vi "NI-XNET Monitor Init.vi"(8 "Error In":errorcluster, 10 "Parameters":variant, 11 "Data Access Engine in":refnum<class "Data Access Engine.lvclass">) -> (0 "Error Out":errorcluster, 3 "Process  Data Out":T1, 4 "Async Loop Rate (s)":dbl)   [LabVIEW 2018, in "NI-XNET Monitor Engine.lvlib"]
uses:
  NI-XNET Monitor Engine.lvlib
  <vilib>/NI/NIVS Inline Async API/_Data Access Engine/Data Access Engine/Data Access Engine.lvclass
  typedefs/RTMonitorRefnums.ctl
  typedefs/CANBus.Settings.ctl
  Bus Load/CANBus/CANBus_Load_Calculator.lvclass
  <vilib>/NI/NIVS Inline Async API/_Data Access Engine/Data Access Engine/Types/Write.DVR.ctl
  <vilib>/NI/NIVS Inline Async API/_Data Access Engine/Access Type Classes/Write/Write.lvclass
  Shared/Compiled.Data.ctl
  Shared/BusLoad.Settings.ctl
  <vilib>/NI/NIVS Inline Async API/_Data Access Engine/Data Access Engine/Methods/Write.Lookup.vi
  Shared/NI-XNET Monitor Shared.lvlib
  <vilib>/NI Veristand/Custom Device Tools/Custom Device Utility Library/Custom Device Utility Library.lvlib
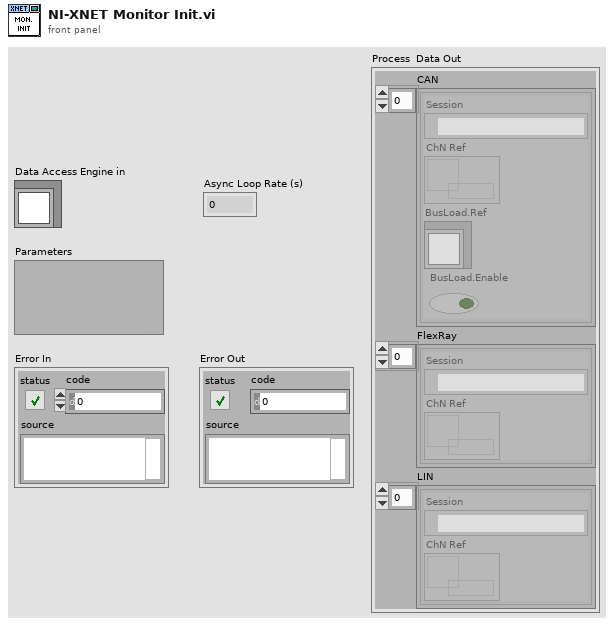
[diagram p1: front panel]
types:
  T1 = typedef "NI-XNET Monitor Engine.lvlib/RTMonitorRefnums.ctl" = cluster{"CAN":T2[], "FlexRay":cluster{"Session":refnum<k21>, "ChN Ref":T3}[], "LIN":cluster{"Session":refnum<k21>, "ChN Ref":T3}[]}
  T2 = typedef "NI-XNET Monitor Engine.lvlib/CANBus.Settings.ctl" = cluster{"Session":refnum<k21>, "ChN Ref":T3, "BusLoad.Ref":refnum<class "CANBus_Load_Calculator.lvclass">, "BusLoad.Enable":bool}
  T3 = typedef "Data Access Engine.lvlib/Data Access Engine.lvclass/Write.DVR.ctl" = refnum<data-value>
  T4 = typedef "NI-XNET Monitor Shared.lvlib/Compiled.Data.ctl" = cluster{"CAN":string[], "FlexRay":string[], "LIN":string[], "Async Loop Rate (s)":dbl, "CAN.BusLoad.Settings":T5[]}
  T5 = typedef "NI-XNET Monitor Shared.lvlib/BusLoad.Settings.ctl" = cluster{"BusLoad.Disable":bool, "BusLoad.Periodms":u32}
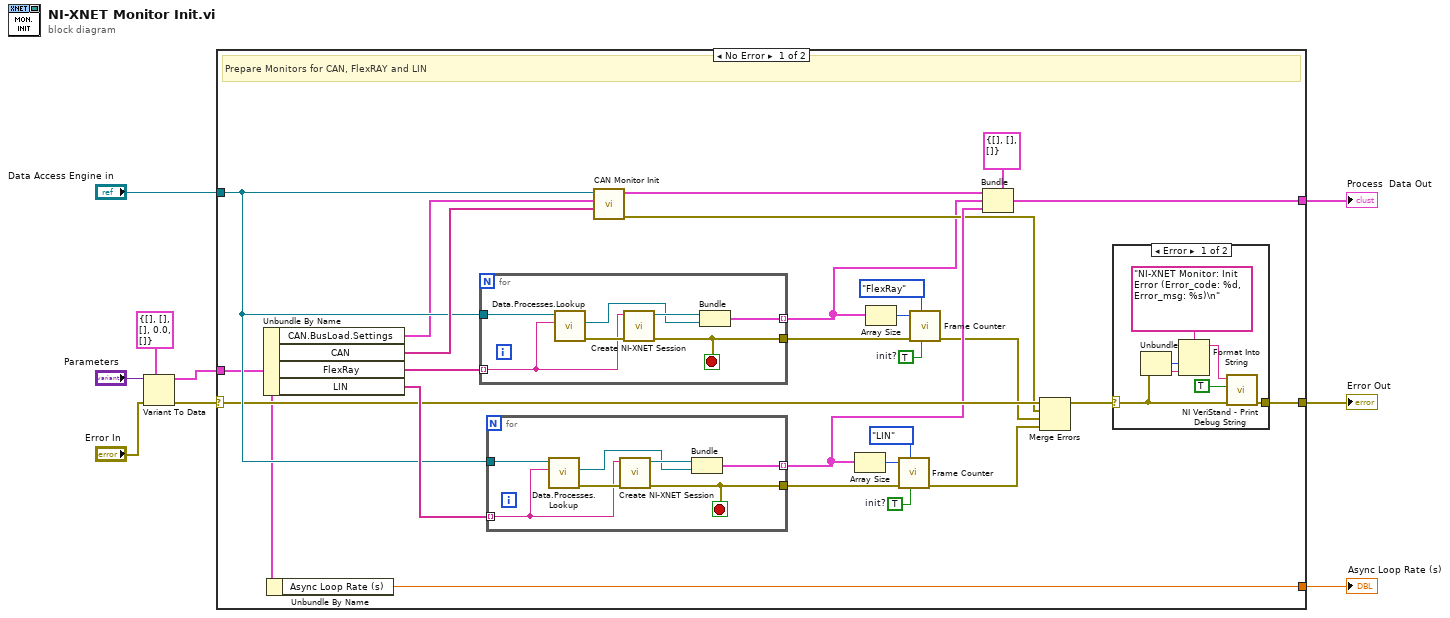
[diagram p0: block diagram]
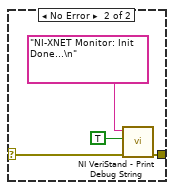
[diagram p2: hidden frame]
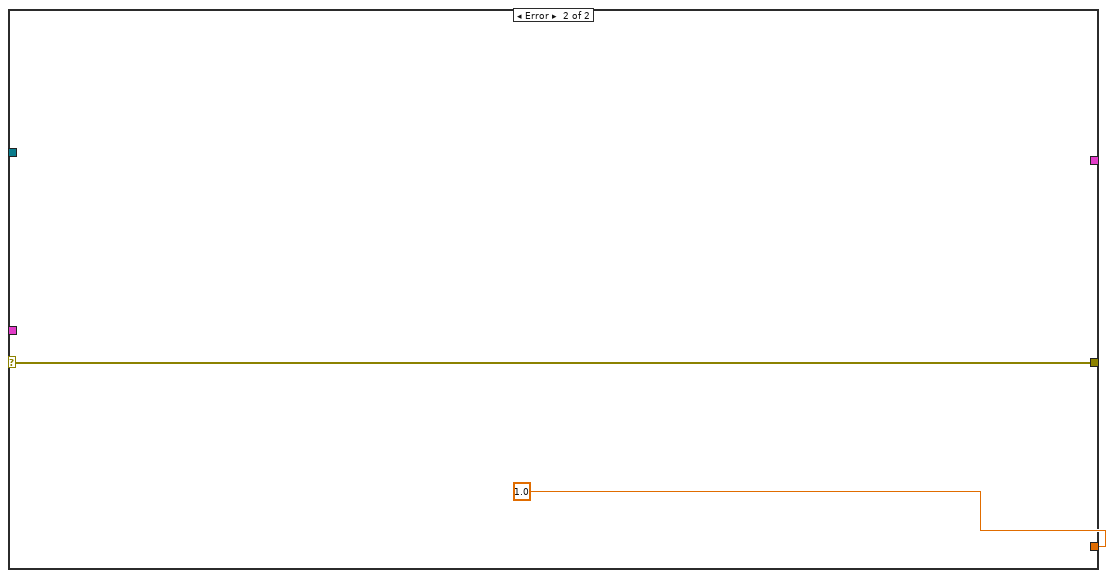
[diagram p3: hidden frame]
diagram:
  n1 = Variant To Data(error in="Error In", type=T4 {"CAN"=[], "FlexRay"=[], "LIN"=[], "Async Loop Rate (s)"=0.0, "CAN.BusLoad.Settings"=[]} ("Compiled.Data"), Variant="Parameters") -> (data=w3:T4, error out=w4:errorcluster)
  n2 = case shown="No Error" w4 {
    selector: w4 -> [w29 w61]
    tunnel: w3 -> [w27 _]
    tunnel: "Data Access Engine in" -> [w31 _]
    tunnel: [w30 _] -> w9
    tunnel: [w24 w61] -> w5
    tunnel: [w26 1.0 ("Async Loop Rate (s)")] -> w1
    frame No Error {
      w16 = TRUE  # init?
      w23 = TRUE  # init?
      # "Prepare Monitors for CAN, FlexRAY and LIN"
      n3 = Unbundle By Name(w27) -> ("CAN.BusLoad.Settings"=w10:T5[], "CAN"=w34:string[], "FlexRay"=w32:string[], "LIN"=w33:string[])
      n4 = Unbundle By Name(w27) -> ("Async Loop Rate (s)"=w26:dbl)
      n5 = for {
        tunnel: w32 -> [w57] mode=indexing
        tunnel: w31 -> [w59]
        tunnel: [w56] -> w15
        tunnel: [w53] -> w11 mode=indexing
        stop <- w56 stop-if-true
        n6 = call-poly <vilib>:"Data.Processes.Lookup.vi"("Name"=w57, "Data Access API in"=w59) -> ("error out"=w58:errorcluster, "Ref"=w54:T3)  [unwired: 6 in, 2 out]
        n7 = call "Create NI-XNET Session.vi"("Error In"=w58, "NI-XNET Port In"=w57) -> ("Error Out"=w56:errorcluster, "Session out"=w55:refnum<k21>)  [unwired: 8 in]
        n8 = Bundle("Session out"=w55, "Ref"=w54) -> (w53:cluster{"Session out":refnum<k21>, "Ref":T3})  [unwired: 1 in]
      }
      n9 = for {
        tunnel: w33 -> [w50] mode=indexing
        tunnel: w31 -> [w52]
        tunnel: [w49] -> w22
        tunnel: [w46] -> w19 mode=indexing
        stop <- w49 stop-if-true
        n10 = call-poly <vilib>:"Data.Processes.Lookup.vi"("Name"=w50, "Data Access API in"=w52) -> ("error out"=w51:errorcluster, "Ref"=w47:T3)  [unwired: 6 in, 2 out]
        n11 = call "Create NI-XNET Session.vi"("Error In"=w51, "NI-XNET Port In"=w50) -> ("Error Out"=w49:errorcluster, "Session out"=w48:refnum<k21>)  [unwired: 8 in]
        n12 = Bundle("Session out"=w48, "Ref"=w47) -> (w46:cluster{"Session out":refnum<k21>, "Ref":T3})  [unwired: 1 in]
      }
      n13 = call "CAN Monitor Init.vi"("CAN Ports"=w34, "CAN.BusLoad.Settings"=w10, "Data Access Engine in"=w31) -> ("error out"=w12:errorcluster, "CAN Runtime Data"=w13:T2[])  [unwired: 7 in]
      n14 = Array Size(array=w19) -> (size(s)=w18:i32)
      n15 = Array Size(array=w11) -> (size(s)=w17:i32)
      n16 = call "Frame Counter.vi"("init? (F)"=w23, "bus type"=enum16{"CAN", "FlexRay", "LIN"}."LIN", "error in (no error)"=w22, "bus index (bus count for init)"=w18) -> ("error out"=w21:errorcluster)  [unwired: 6 in, 1 out]
      n17 = call "Frame Counter.vi"("init? (F)"=w16, "bus type"=enum16{"CAN", "FlexRay", "LIN"}."FlexRay", "error in (no error)"=w15, "bus index (bus count for init)"=w17) -> ()  [unwired: 6 in, 2 out]
      n18 = Bundle(cluster=T1 {"CAN"=[], "FlexRay"=[], "LIN"=[]}, "CAN"=w13, "FlexRay"=w11, "LIN"=w19) -> (w30:T1)
      n19 = Merge Errors(w29, w12, w15, w21) -> (w25:errorcluster)
      n20 = case shown="Error" w25 {
        selector: w25 -> [w36 w44]
        tunnel: [w35 w43] -> w24
        frame Error {
          n21 = Unbundle(w36) -> ("code"=w40:i32, "source"=w41:string)  [unwired: 1 out]
          n22 = Format Into String(format string="NI-XNET Monitor: Init Error (Error_code: %d, Error_msg: %s)\n" ("Message"), w40, w41) -> (resulting string=w39:string)  [unwired: 2 in, 1 out]
          n23 = call <vilib>:"NI VeriStand - Print Debug String.vi"("error in (no error)"=w36, "Add to log file? (T)"=TRUE, "Message"=w39) -> ("error out"=w35:errorcluster)  [unwired: 8 in]
        }
        frame No Error {
          n24 = call <vilib>:"NI VeriStand - Print Debug String.vi"("error in (no error)"=w44, "Add to log file? (T)"=TRUE, "Message"="NI-XNET Monitor: Init Done...\n") -> ("error out"=w43:errorcluster)  [unwired: 8 in]
        }
      }
    }
    frame Error {
    }
  }
  "Error Out" <- w5
  "Process  Data Out" <- w9
  "Async Loop Rate (s)" <- w1
